vi "move_stp_Motion.vi"(8 "error in (no error)":errorcluster caption="错误输入（无错误）", 10 "stp":dbl min=0.0, 11 "OneMotion 输入":refnum<class "OneMotion.lvclass">) -> (0 "error out":errorcluster caption="错误输出", 3 "OneMotion 输出":refnum<class "OneMotion.lvclass">)   [LabVIEW 2016, in "MotionControl.lvlib" / "OneMotion.lvclass"]
uses:
  <userlib>/MotionControl/OneMotion/OneMotion.lvclass
  <userlib>/MotionControl/OneMotion/OneMotion.lvclass/OneMotion.ctl
  <userlib>/MotionControl/StepMotor/StepMotor.lvclass
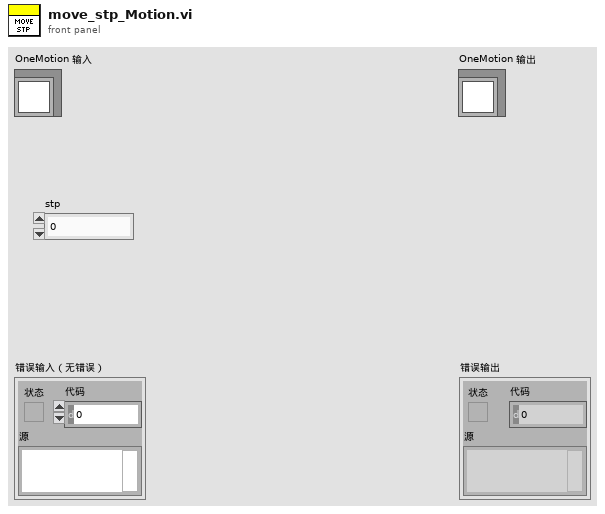
[diagram p1: front panel]
types:
  T1 = typedef "MotionControl.lvlib/OneMotion.lvclass/unit mode.ctl" = enum16{"motor (pulse)", "linear (mm) or radial (degree)"}
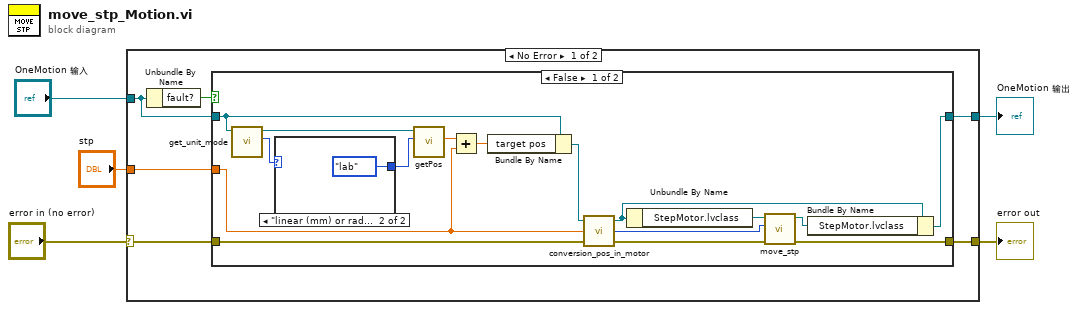
[diagram p0: block diagram]
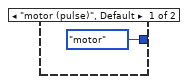
[diagram p2: hidden frame]
diagram:
  n1 = case shown="No Error" "error in (no error)" {
    selector: "error in (no error)" -> [w11 w33]
    tunnel: [w10 w33] -> w3
    tunnel: [w9 w32] -> w2
    tunnel: "OneMotion 输入" -> [w8 w32]
    tunnel: "stp" -> [w6 _]
    frame No Error {
      n2 = Unbundle By Name(w8) -> ("fault?"=w7:bool)
      n3 = case shown="False" w7 {
        tunnel: w11 -> [w27 w30]
        tunnel: [w21 w30] -> w10
        tunnel: w6 -> [w13 _]
        tunnel: [w24 w31] -> w9
        tunnel: w8 -> [w18 w31]
        frame False {
          n4 = call-dynamic "get_unit_mode.vi"("OneMotion输入"=w18) -> ("unit mode"=w16:T1, "OneMotion输出"=w17:refnum<class "OneMotion.lvclass">)  [unwired: 8 in, 1 out]
          n5 = case shown="\"linear (mm) or radial (degree)\"" w16 {
            tunnel: [enum16{"lab", "motor"}."motor" ("lab or motor") enum16{"lab", "motor"}."lab" ("lab or motor")] -> w15
            frame "motor (pulse)", Default {
            }
            frame "linear (mm) or radial (degree)" {
            }
          }
          n6 = call <userlib>:"getPos.vi"("lab or motor"=w15, "OneMotion 输入"=w17) -> ("pos"=w14:dbl)  [unwired: 7 in, 2 out]
          n7 = Add(x=w14, y=w13) -> (x+y=w12:dbl)
          n8 = Bundle By Name(cluster=w18, "target pos"=w12) -> (w25:refnum<class "OneMotion.lvclass">)
          n9 = call <userlib>:"conversion_pos_in_motor.vi"("error in (no error)"=w27, "pos"=w13, "OneMotion 输入"=w25) -> ("error out"=w22:errorcluster, "pos in motor"=w19:i32, "OneMotion 输出"=w26:refnum<class "OneMotion.lvclass">)
          n10 = Unbundle By Name(w26) -> ("StepMotor.lvclass"=w23:refnum<class "StepMotor.lvclass">)
          n11 = call <userlib>:"move_stp.vi"("error in (no error)"=w22, "stp"=w19, "StepMotor 输入"=w23) -> ("error out"=w21:errorcluster, "StepMotor 输出"=w20:refnum<class "StepMotor.lvclass">)  [unwired: 7 in]
          n12 = Bundle By Name(cluster=w26, "StepMotor.lvclass"=w20) -> (w24:refnum<class "OneMotion.lvclass">)
        }
        frame True {
        }
      }
    }
    frame Error {
    }
  }
  "error out" <- w3
  "OneMotion 输出" <- w2
